vi "readQRcode.vi"(1 "error out":errorcluster, 8 "stop":bool=TRUE, 9 "New Image":T1, 11 "Session Out":T2) -> (0 "Start Out Point":dbl[](array[numeric])=[0.0, 0.1725], 2 "Image":T1(plugin-control), 3 "X/Y/Z":dbl[](array[numeric]), 4 "Start Front":dbl[](array[numeric])=[0.0, 0.3925, 0.0], 5 "Start POS":dbl[](array[numeric]), 6 "Block Array":dbl[][](array[numeric]), 7 "heading":dbl)   [LabVIEW 2018]
uses:
  <vilib>/userdefined/High Color/IMAQdx.ctl
  <vilib>/vision/Image Controls.llb/IMAQ Image.ctl
  22485c95-b937-49fe-bc35-04f8ff6dd2f9.vi
  <vilib>/Analysis/coordinate.llb/2D Cartesian Coordinate Rotation (Scalar).vi
  <vilib>/Array/Sort 2D Array - Pop Stack.vi
  <vilib>/Array/Sort 2D Array - Push Stack.vi
  22485c95-b937-49fe-bc35-04f8ff6dd2f9.vi/fce0ab3c-cf09-405a-b55b-6ad9e4deb79f.vi
  22485c95-b937-49fe-bc35-04f8ff6dd2f9.vi/4c1c8537-9a2a-4327-8778-8b4582560b89.vi
  <vilib>/Analysis/NI_AALPro.lvlib
panel:
  out "QR_CODE":string="(K,Q,J,N)(I,I,K,G)(N,C,P,E)(E,O,C,Q)"
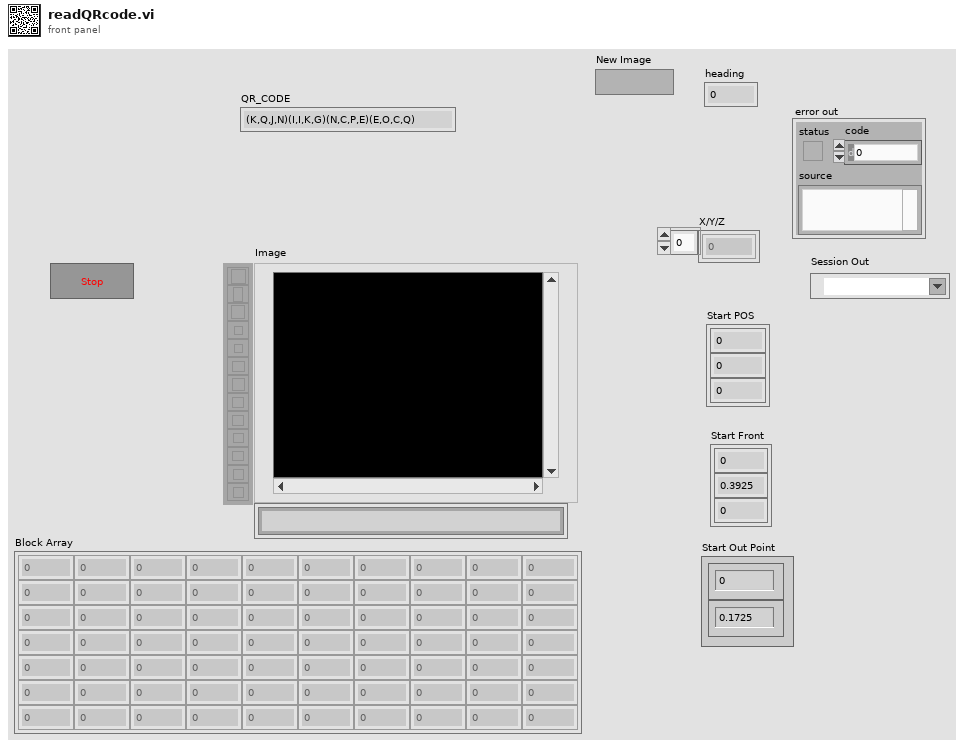
[diagram p1: front panel]
types:
  T1 = typedef "IMAQ Image.ctl" = refnum<image>
  T2 = typedef "IMAQdx.ctl" = refnum<k21>
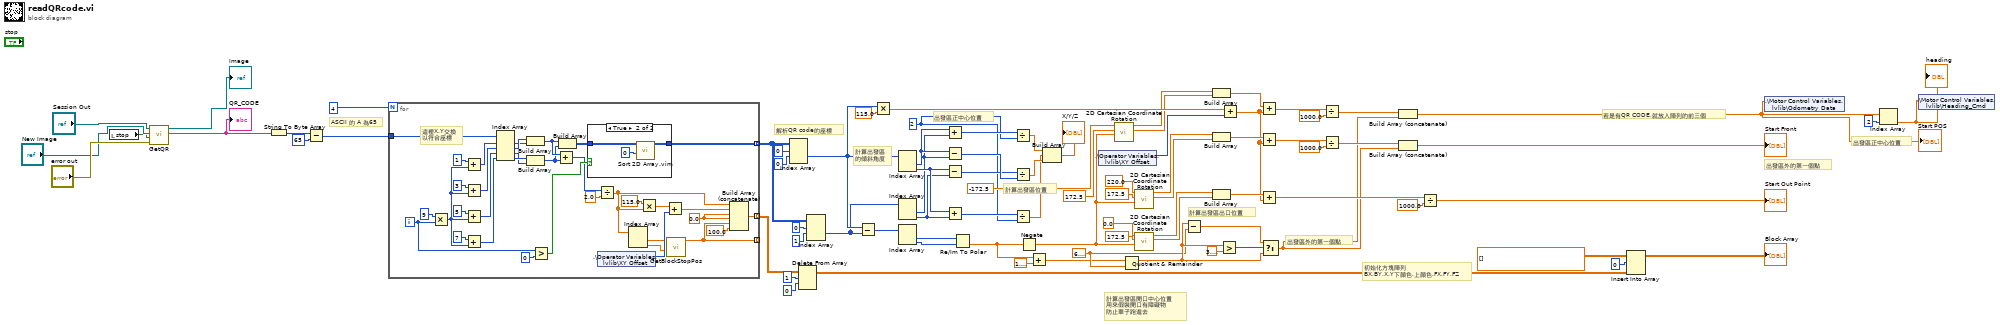
[diagram p0: block diagram]
diagram:
  w10 = 2 ("y")
  w70 = 6.283185307179586
  # "若是有QR CODE,就放入陣列的前三個"
  # "計算出發區開口中心位置\n用來假裝開口有障礙物\n防止車子跑進去"
  # "出發區外的第一個點"
  # "出發區正中心位置"
  # "初始化方塊陣列\nBX,BY,X,Y下顏色,上顏色,FX,FY,FZ"
  # "出發區外的第一個點"
  # "出發區正中心位置"
  # "計算出發區出口位置"
  # "計算出發區位置"
  # "計算出發區\n的傾斜角度"
  # "解析QR code的座標"
  # "ASCII 的 A 為65"
  n1 = local read "stop"() -> (w1:bool)
  n2 = call "GetQR.vi"("error in"="error out", "STOP"=w1, "Image In"="New Image", "Session In"="Session Out") -> ("QR_CODE"=w36:string, "Image Out"=→"Image":T1)  [unwired: 5 in, 1 out]
  "QR_CODE" <- w36
  n3 = String To Byte Array(string=w36) -> (unsigned byte array=w51:u8[])
  n4 = Subtract(x=w51, y=65) -> (x-y=w53:i32[])
  n5 = for {
    N: 4 -> [_]
    tunnel: w53 -> [w117]
    tunnel: [w106] -> w57 mode=indexing
    tunnel: [w85] -> _ mode=indexing
    tunnel: [w83] -> w27 mode=indexing
    i -> [w104]
    w89 = 0.0
    # "這裡X,Y交換\n以符合座標"
    n6 = Multiply(x=9, y=w104) -> (x*y=w111:i32)
    n7 = Add(x=1 ("index"), y=w111) -> (x+y=w110:i32)
    n8 = Add(x=3 ("index"), y=w111) -> (x+y=w109:i32)
    n9 = Add(x=5 ("index"), y=w111) -> (x+y=w108:i32)
    n10 = Add(x=7 ("index"), y=w111) -> (x+y=w107:i32)
    n11 = Index Array(array=w117, index #1=w110, index #2=w109, index #3=w108, index #4=w107) -> (element #1=w100:i32, element #2=w101:i32, element #3=w98:i32, element #4=w99:i32)
    n12 = Build Array(w101, w100) -> (w97:i32[])
    n13 = Build Array(w99, w98) -> (w94:i32[])
    n14 = Greater?(x=w104, y=0) -> (0:w105:bool)
    n15 = Add(x=w97, y=w94) -> (x+y=w96:i32[])
    n16 = Build Array(w97, w94) -> (w102:i32[][])
    n17 = case shown="True" w105 {
      tunnel: w102 -> [w118 w121]
      tunnel: [w118 w119] -> w106
      frame False {
      }
      frame True {
        n18 = call "Sort 2D Array.vim"("index"=0, "2D array"=w121) -> ("sorted 2D array"=w119:i32[][])  [unwired: 8 in, 1 out]
      }
    }
    n19 = shared-variable ".\\Operator Variables.lvlib\\XY Offset"() -> (w90:i16)  [unwired: 1 in, 1 out]
    n20 = Divide(x=w96, y=2.0) -> (x/y=w84:dbl[])
    n21 = Index Array(array=w84) -> (element #1=w87:dbl, element #2=w86:dbl)  [unwired: 2 in]
    n22 = Multiply(x=115.0, y=w84) -> (x*y=w91:dbl[])
    n23 = Add(x=w91, y=w90) -> (x+y=w92:dbl[])
    n24 = call "GetBlockStopPos.vi"("YB"=w86, "XB"=w87) -> ("Array"=w85:dbl[])  [unwired: 8 in, 1 out]
    n25 = Build Array (concatenate)(w84, w92, w89, w89, w85, 100.0) -> (w83:dbl[])
  }
  n26 = Index Array(array=w57, index (dim 0)=0 ("index (page)"), index (dim 1)=0 ("disabled index (row)")) -> (element=w21:i32[])  [unwired: 1 in]
  n27 = Delete From Array(array=w27, length=1, index (row)=0) -> (array with subset deleted=w32:dbl[][])  [unwired: 1 in, 1 out]
  n28 = Index Array(array=w57, index (dim 0)=0 ("index (page)"), index (dim 1)=1 ("disabled index (row)")) -> (element=w20:i32[])  [unwired: 1 in]
  n29 = Subtract(x=w21, y=w20) -> (x-y=w60:i32[])
  n30 = Multiply(x=w21, y=115.0) -> (x*y=w75:dbl[])
  n31 = Index Array(array=w21) -> (element #1=w16:i32, element #2=w15:i32)  [unwired: 2 in]
  n32 = Index Array(array=w20) -> (element #1=w14:i32, element #2=w13:i32)  [unwired: 2 in]
  n33 = Index Array(array=w60) -> (element #1=w61:i32, element #2=w62:i32)  [unwired: 2 in]
  n34 = Add(x=w16, y=w14) -> (x+y=w12:i32)
  n35 = Subtract(x=w16, y=w14) -> (x-y=w19:i32)
  n36 = Subtract(x=w15, y=w13) -> (x-y=w18:i32)
  n37 = Add(x=w15, y=w13) -> (x+y=w11:i32)
  n38 = Re/Im To Polar(2:w62, 3:w61) -> (0:w82:dbl)  [unwired: 1 out]
  n39 = Divide(x=w12, y=w10) -> (x/y=w8:dbl)
  n40 = Divide(x=w18, y=w19) -> (x/y=w7:dbl)
  n41 = Divide(x=w11, y=w10) -> (x/y=w6:dbl)
  n42 = Negate(x=w82) -> (-x=w41:dbl)
  n43 = Add(x=w82, y=1.5707963267948966) -> (x+y=w66:dbl)
  n44 = Build Array(w8, w6, w7) -> (→"X/Y/Z":dbl[])
  n45 = shared-variable ".\\Operator Variables.lvlib\\XY Offset"() -> (w76:i16)  [unwired: 1 in, 1 out]
  n46 = call-poly <vilib>:"2D Cartesian Coordinate Rotation.vi"("theta"=w41, "y"=172.5, "x"=-172.5) -> ("y out"=w73:dbl, "x out"=w72:dbl)  [unwired: 6 in, 1 out]
  n47 = Quotient & Remainder(x=w66, y=w70) -> (x-y*floor(x/y)=w71:dbl)  [unwired: 1 out]
  n48 = call-poly <vilib>:"2D Cartesian Coordinate Rotation.vi"("theta"=w41, "y"=172.5, "x"=220.0) -> ("y out"=w80:dbl, "x out"=w79:dbl)  [unwired: 6 in, 1 out]
  n49 = call-poly <vilib>:"2D Cartesian Coordinate Rotation.vi"("theta"=w41, "y"=172.5, "x"=0.0) -> ("y out"=w43:dbl, "x out"=w44:dbl)  [unwired: 6 in, 1 out]
  n50 = Subtract(x=w71, y=w70) -> (x-y=w69:dbl)
  n51 = Build Array(w72, w73) -> (w74:dbl[])
  n52 = Build Array(w79, w80) -> (w81:dbl[])
  n53 = Build Array(w44, w43) -> (w40:dbl[])
  n54 = Greater?(x=w71, y=3.141592653589793) -> (0:w68:bool)
  n55 = Add(x=w75, y=w76) -> (x+y=w39:dbl[])
  n56 = Add(x=w74, y=w39) -> (x+y=w47:dbl[])
  n57 = Add(x=w81, y=w39) -> (x+y=w49:dbl[])
  n58 = Add(x=w40, y=w39) -> (x+y=w38:dbl[])
  n59 = Select(t=w69, s=w68, f=w71) -> (s? t:f=w35:dbl)
  n60 = Divide(x=w47, y=1000.0) -> (x/y=w17:dbl[])
  n61 = Divide(x=w49, y=1000.0) -> (x/y=w48:dbl[])
  n62 = Build Array (concatenate)(w17, w35) -> (w25:dbl[])
  "Start POS" <- w25
  n63 = Build Array (concatenate)(w48, w35) -> (→"Start Front":dbl[])
  n64 = Divide(x=w38, y=1000.0) -> (x/y=→"Start Out Point":dbl[])
  n65 = Insert Into Array(array=dbl[][] [], index (row)=0, new element=w32) -> (→"Block Array":dbl[][])  [unwired: 1 in]
  n66 = shared-variable ".\\Motor Control Variables.lvlib\\Odometry Data"(w25) -> ()  [unwired: 1 in, 1 out]
  n67 = Index Array(array=w25, index=2) -> (element=w23:dbl)
  "heading" <- w23
  n68 = shared-variable ".\\Motor Control Variables.lvlib\\Heading_Cmd"(w23) -> ()  [unwired: 1 in, 1 out]
